vi "makeDecisions.vi"(8 "error in (no error)":errorcluster, 10 "model":refnum<class "Model.lvclass">, 11 "MovingToNewForceState in":refnum<class "RequestingNewSetpointState.lvclass">) -> (0 "error out":errorcluster, 2 "model 2":refnum<class "Model.lvclass">, 3 "MovingToNewForceState out":refnum<class "RequestingNewSetpointState.lvclass">)   [LabVIEW 2013, in "RequestingNewSetpointState.lvclass"]
uses:
  RequestingNewSetpointState.lvclass
  Model/Model/Model.lvclass
  Typedefs/StateSelector.ctl
  MovingToNewTemperatureState/MovingToNewTemperatureState.lvclass
  Typedefs/AITDTTypedefs.lvlib
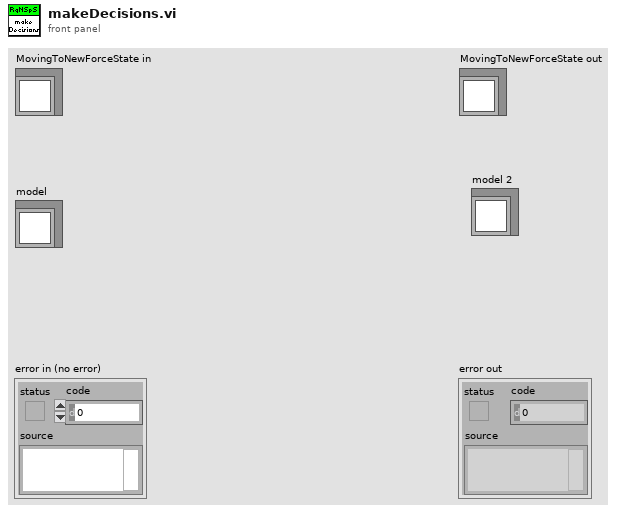
[diagram p1: front panel]
types:
  T1 = typedef "AITDTTypedefs.lvlib/StateSelector.ctl" = enum16{"AwaitingSetpointAcknowledgmentState", "EndingCycleState", "FaultState", "OffState", "PausingState", "RequestingNewSetpointState", "SamplingState", "SettlingState", "SoakingState", "StabilizingState", "StandbyState", "StoppedState", "TransitioningTemperatureState"}
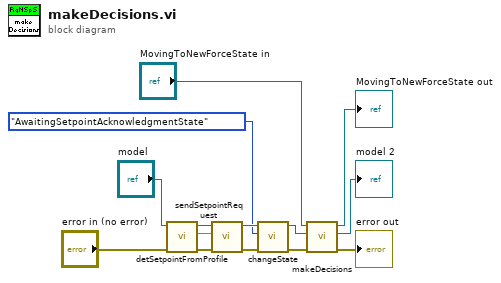
[diagram p0: block diagram]
diagram:
  n1 = call "detSetpointFromProfile.vi"("error in (no error)"="error in (no error)", "Model in"="model") -> ("error out"=w2:errorcluster, "temperatureSetpoint"=w3:dbl[unit], "Model out"=w4:refnum<class "Model.lvclass">)  [unwired: 7 in]
  n2 = call "sendSetpointRequest.vi"("error in (no error)"=w2, "temperatureSetpoint"=w3, "Model in"=w4) -> ("error out"=w8:errorcluster, "Model out"=w10:refnum<class "Model.lvclass">)  [unwired: 7 in]
  n3 = call "changeState.vi"("error in (no error)"=w8, "State:"=StateSelector."AwaitingSetpointAcknowledgmentState", "Model in"=w10) -> ("error out"=w7:errorcluster, "Model out"=w6:refnum<class "Model.lvclass">)  [unwired: 7 in]
  n4 = call-parent "makeDecisions.vi"("error in (no error)"=w7, "model"=w6, "EnabledState in"="MovingToNewForceState in") -> ("error out"=→"error out":errorcluster, "model 2"=→"model 2":refnum<class "Model.lvclass">, "EnabledState out"=→"MovingToNewForceState out":refnum<class "RequestingNewSetpointState.lvclass">)  [unwired: 6 in]
